vi "Set Scope Mode.vi"(8 "error in (no error)":errorcluster, 10 "Scope Mode (0: Off)":u32(ring) items=["Off", "AC & DC Voltage", "Edge", "Leveled Sine", "Marker", "Wave Generator", "Video", "Pulse", "Impedance & Capacitance Meas", "Overload"], 11 "VISA resource name":refnum<visa-resource-name>) -> (0 "error out":errorcluster {"code" format="%.0x"}, 3 "VISA resource name out":refnum<visa-resource-name>)   [LabVIEW 2014, in "Fluke 5XXX Series Multicalibrators.lvlib"]
doc: "This VI sets the oscilloscope’s mode of operation.\n\nOnce in SCOPE mode, use the FL5XMCAL Set Output Values.vi to program new output in all VIs except FL5XMCAL Impedance Measurement.vi and the FL5XMCAL Set Calibrator Range.vi as required (in OVERLD, PULSE, and MEAS Z functions only.)\n\nThe FL5XMCAL Get Function Type.vi returns the corresponding oscilloscope modes.\n\nNote:\n\nThis VI is available only for instrument models 5500A and 5520A with oscilloscope option SC300 (SC600 or SC1100)."
uses:
  Fluke 5XXX Series Multicalibrators.lvlib
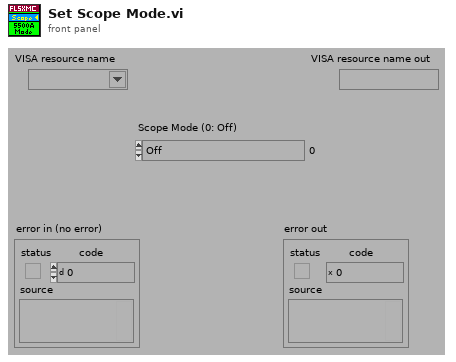
[diagram p1: front panel]
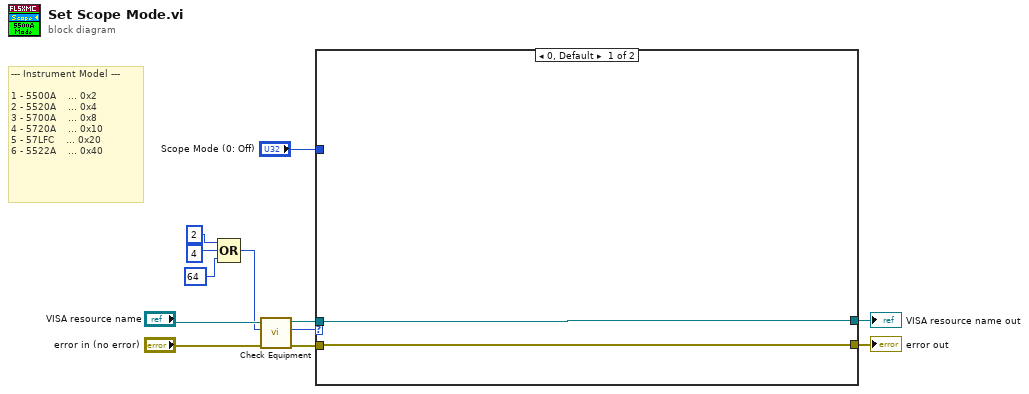
[diagram p0: block diagram]
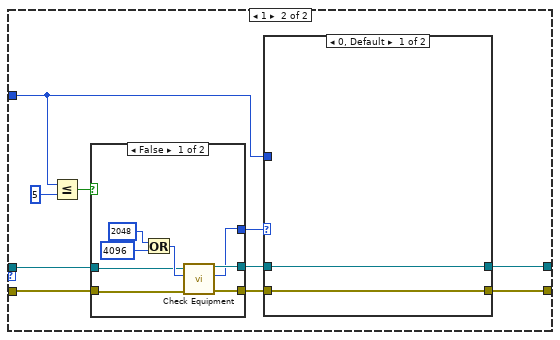
[diagram p2: hidden frame]
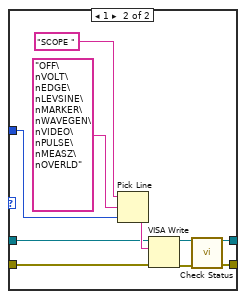
[diagram p3: hidden frame]
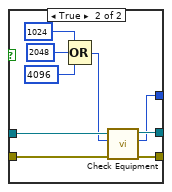
[diagram p4: hidden frame]
diagram:
  # "--- Instrument Model ---\n\n1 - 5500A    ... 0x2\n2 - 5520A    ... 0x4\n3 - 5700A    ... 0x8\n4 - 5720A    ... 0x10\n5 - 57LFC    ... 0x20\n6 - 5522A    ... 0x40"
  n1 = Compound Arithmetic op=OR(2 ("Numeric"), 4 ("Numeric"), 64 ("Numeric")) -> (w4:i32)
  n2 = call "Check Equipment.vi"("error in (no error)"="error in (no error)", "Bit Mask"=w4, "VISA resource name"="VISA resource name") -> ("error out"=w12:errorcluster, "Present?"=w5:u32, "VISA resource name out"=w11:refnum<visa-resource-name>)  [unwired: 6 in]
  n3 = case shown="0, Default" w5 {
    tunnel: "Scope Mode (0: Off)" -> [_ w22]
    tunnel: [w13 w23] -> w7
    tunnel: w12 -> [w14 w19]
    tunnel: w11 -> [w13 w18]
    tunnel: [w14 w24] -> w6
    frame 0, Default {
    }
    frame 1 {
      n4 = Less Or Equal?(x=w22, y=u32 5) -> (x <= y?=w20:bool)
      n5 = case shown="False" w20 {
        tunnel: w19 -> [w39 w53]
        tunnel: w18 -> [w40 w52]
        tunnel: [w42 w51] -> w17
        tunnel: [w41 w50] -> w16
        tunnel: [w37 w45] -> w15
        frame False {
          n6 = Or(x=2048 ("Numeric"), y=4096 ("Numeric")) -> (x .or. y?=w44:i32)
          n7 = call "Check Equipment.vi"("error in (no error)"=w39, "Bit Mask"=w44, "VISA resource name"=w40) -> ("error out"=w42:errorcluster, "Present?"=w37:u32, "VISA resource name out"=w41:refnum<visa-resource-name>)  [unwired: 6 in]
        }
        frame True {
          n8 = Compound Arithmetic op=OR(1024 ("Numeric"), 2048 ("Numeric"), 4096 ("Numeric")) -> (w46:i32)
          n9 = call "Check Equipment.vi"("error in (no error)"=w53, "Bit Mask"=w46, "VISA resource name"=w52) -> ("error out"=w51:errorcluster, "Present?"=w45:u32, "VISA resource name out"=w50:refnum<visa-resource-name>)  [unwired: 6 in]
        }
      }
      n10 = case shown="0, Default" w15 {
        tunnel: [w25 w27] -> w24
        tunnel: [w26 w31] -> w23
        tunnel: w22 -> [_ w30]
        tunnel: w17 -> [w25 w29]
        tunnel: w16 -> [w26 w28]
        frame 0, Default {
        }
        frame 1 {
          n11 = Pick Line(string ("")="SCOPE " ("Reset Command"), multi-line string="OFF\nVOLT\nEDGE\nLEVSINE\nMARKER\nWAVEGEN\nVIDEO\nPULSE\nMEASZ\nOVERLD", line index=w30) -> (output string=w34:string)
          n12 = VISA Write(VISA resource name=w28, write buffer=w34, error in (no error)=w29) -> (VISA resource name out=w32:refnum<visa-resource-name>, error out=w33:errorcluster)  [unwired: 1 out]
          n13 = call "Check Status.vi"("VISA resource name"=w32, "error in (no error)"=w33) -> ("VISA resource name out"=w31:refnum<visa-resource-name>, "error out"=w27:errorcluster)  [unwired: 12 in]
        }
      }
    }
  }
  "VISA resource name out" <- w7
  "error out" <- w6
